vi "START ADD ITEM.vi"(10 "REFERENCES":T2, 11 "ITEM DATA IN":T1) -> (3 "ITEM DATA OUT":T1)   [LabVIEW 2019]
uses:
  Controls/References Cluster.ctl
  <vilib>/userDefined/High Color/IMAQdx.ctl
  Controls/Custom Calendar/Custom Calendar.xctl
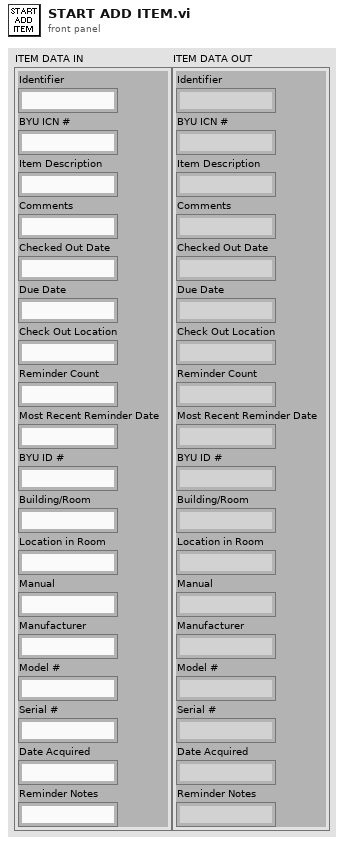
[diagram p1: front panel]
types:
  T1 = cluster{"Identifier":string, "BYU ICN #":string, "Item Description":string, "Comments":string, "Checked Out Date":string, "Due Date":string, "Check Out Location":string, "Reminder Count":string, "Most Recent Reminder Date":string, "BYU ID #":string, "Building/Room":string, "Location in Room":string, "Manual":string, "Manufacturer":string, "Model #":string, "Serial #":string, "Date Acquired":string, "Reminder Notes":string}
  T2 = typedef "References Cluster.ctl" = cluster{"MAIN PAGES":refnum<vi>, "ADD/EDIT ITEM REFERENCES":cluster{"Identifier":refnum<vi>, "BYU ICN #":refnum<vi>, "Item Description":refnum<vi>, "Comments":refnum<vi>, "Checked Out Date":refnum<vi>, "Due Date":refnum<vi>, "Check Out Location":refnum<vi>, "Reminder Count":refnum<vi>, "Most Recent Reminder Date":refnum<vi>, "BYU ID #":refnum<vi>, "Building/Room":refnum<vi>, "Location in Room":refnum<vi>, "Manual":refnum<vi>, "Manufacturer":refnum<vi>, "Model #":refnum<vi>, "Serial #":refnum<vi>, "Date Acquired":refnum<vi>, "ADD/EDIT ITEM LABEL":refnum<vi>, "ARCHIVE ITEM":refnum<vi>, "Archive Item Inputs":refnum<vi>, "Reminder Notes":refnum<vi>, "DUPLICATE ITEM":refnum<vi>}, "ADD/EDIT USER REFERENCES":cluster{"BYU ID # (##-###-####)":refnum<vi>, "First Name":refnum<vi>, "Last Name":refnum<vi>, "Phone Number (###-###-####)":refnum<vi>, "Email":refnum<vi>, "Department":refnum<vi>, "Graduation Status":refnum<vi>, "Anticipated Graduation Year":refnum<vi>, "Credit Score":refnum<vi>, "Date Added":refnum<vi>, "Graduation Clearance Date":refnum<vi>, "Picture File Name":refnum<vi>, "ADD/EDIT USER LABEL":refnum<vi>, "Department Map":refnum<vi>, "Status Map":refnum<vi>, "Anticipated Graduation Year Map":refnum<vi>, "User Agreement":refnum<vi>, "User Comments":refnum<vi>, "Camera":refnum<vi>}, "RETURN ITEM REFERENCES":cluster{"Item or Person:":refnum<vi>, "Search Return Results":refnum<vi>, "What are you searching for?":refnum<vi>}, "SEARCH DATABASE REFERENCES":cluster{"What to Search For:":refnum<vi>, "Where to Search":refnum<vi>, "Column to Search In":refnum<vi>, "Column to Sort By":refnum<vi>, "Search Database Results":refnum<vi>, "Inventory Column Selector":refnum<vi>, "User Column Selector":refnum<vi>, "Inventory Archive Column Selector":refnum<vi>, "User Archive Column Selector":refnum<vi>, "Sales Tracking Column Selector":refnum<vi>, "Checked In Archive Column Selector":refnum<vi>, "Restore User":refnum<vi>, "Date Range":refnum<vi>, "Dates Less Than":refnum<vi>, "Dates Greater Than":refnum<vi>, "Search Print Receipt":refnum<vi>, "Edit Sale Description":refnum<vi>}, "USER ITEMS REFERENCES":cluster{"USER'S INFORMATION":refnum<vi>, "User's Checked Out Items":refnum<vi>, "User Info Comments":refnum<vi>, "SEE USER INFO COMMENTS":refnum<vi>}, "EDIT ITEMS REFERENCES":cluster{"New Check Out Location":refnum<vi>, "Items to Edit":refnum<vi>, "Edit Items Due Date":refnum<vi>, "New Reminder Notes":refnum<vi>, "New Item Description":refnum<vi>}, "CHECK OUT ITEMS REFERENCES":cluster{"Enter Item:":refnum<vi>, "Check Out Items Due Date":refnum<vi>, "Check Out Location":refnum<vi>, "Items to be Checked Out":refnum<vi>, "Possible Items":refnum<vi>, "Altered Item Description":refnum<vi>}, "TRANSFER ITEMS REFERENCES":cluster{"Search Parameter":refnum<vi>, "What to Match":refnum<vi>, "Matching Individuals":refnum<vi>, "Items to be Transferred":refnum<vi>}, "SETTINGS REFERENCES":cluster{"PSC Database Settings":refnum<vi>, "PSC Sales Item Spreadsheet":refnum<vi>}, "PSC SALES REFERENCES":cluster{"BYU ID CARD #":refnum<vi>, "Sale Description":refnum<vi>, "Scan or Enter Item Name":refnum<vi>, "Items to be Sold":refnum<vi>, "Grand Total":refnum<vi>, "Item List":refnum<vi>}}
  T3 = enum32{"IDLE", "ADD/EDIT USER", "ADD/EDIT ITEM", "RETURN ITEMS", "SEARCH DATABASE", "USER ITEMS", "CHECK OUT ITEMS", "EDIT ITEMS", "TRANSFER ITEMS", "PSC SALES", "ATRIUM", "INVENTORY TRACKING", "SETTINGS"}
  T4 = cluster{"Identifier":refnum<vi>, "BYU ICN #":refnum<vi>, "Item Description":refnum<vi>, "Comments":refnum<vi>, "Checked Out Date":refnum<vi>, "Due Date":refnum<vi>, "Check Out Location":refnum<vi>, "Reminder Count":refnum<vi>, "Most Recent Reminder Date":refnum<vi>, "BYU ID #":refnum<vi>, "Building/Room":refnum<vi>, "Location in Room":refnum<vi>, "Manual":refnum<vi>, "Manufacturer":refnum<vi>, "Model #":refnum<vi>, "Serial #":refnum<vi>, "Date Acquired":refnum<vi>, "ADD/EDIT ITEM LABEL":refnum<vi>, "ARCHIVE ITEM":refnum<vi>, "Archive Item Inputs":refnum<vi>, "Reminder Notes":refnum<vi>, "DUPLICATE ITEM":refnum<vi>}
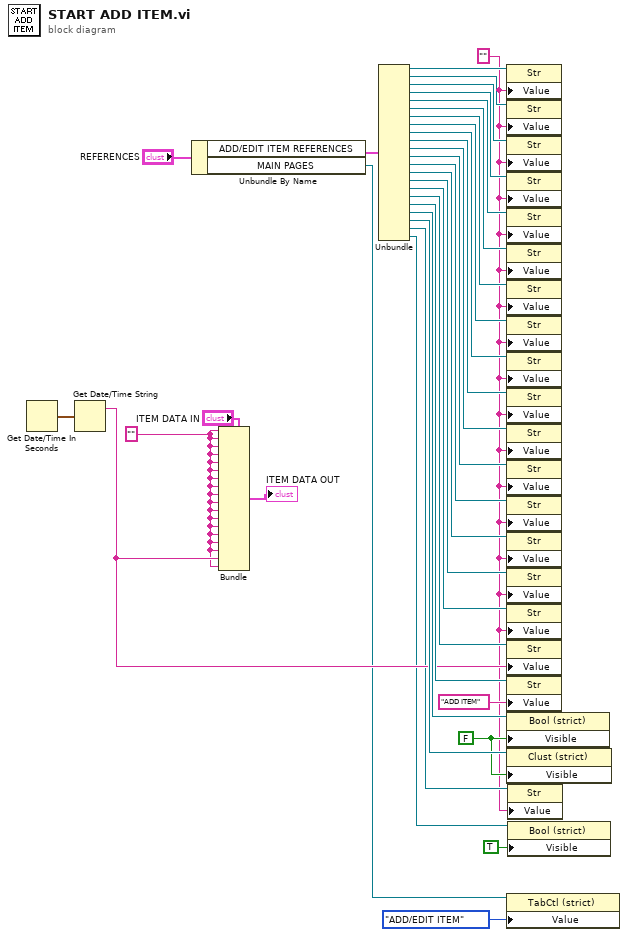
[diagram p0: block diagram]
diagram:
  w13 = FALSE ("Visible")
  w5 = "" ("BYU ID (##-###-####)")
  w3 = "" ("BYU ID (##-###-####)")
  n1 = Get Date/Time In Seconds() -> (seconds since 1Jan1904=w35:timestamp)
  n2 = Get Date/Time String(seconds (now)=w35) -> (date string=w8:string)  [unwired: 2 in, 1 out]
  n3 = Unbundle By Name("REFERENCES") -> ("ADD/EDIT ITEM REFERENCES"=w11:T4, "MAIN PAGES"=w7:refnum<vi>)
  n4 = Bundle(cluster="ITEM DATA IN", "Identifier"=w5, "BYU ICN #"=w5, "Item Description"=w5, "Comments"=w5, "Checked Out Date"=w5, "Due Date"=w5, "Check Out Location"=w5, "Reminder Count"=w5, "Most Recent Reminder Date"=w5, "BYU ID #"=w5, "Building/Room"=w5, "Location in Room"=w5, "Manual"=w5, "Manufacturer"=w5, "Model #"=w5, "Serial #"=w5, "Date Acquired"=w8, "Reminder Notes"=w5) -> (→"ITEM DATA OUT":T1)
  n5 = Unbundle(w11) -> ("Identifier"=w34:refnum<vi>, "BYU ICN #"=w33:refnum<vi>, "Item Description"=w32:refnum<vi>, "Comments"=w31:refnum<vi>, "Checked Out Date"=w30:refnum<vi>, "Due Date"=w29:refnum<vi>, "Check Out Location"=w28:refnum<vi>, "Reminder Count"=w27:refnum<vi>, "Most Recent Reminder Date"=w26:refnum<vi>, "BYU ID #"=w25:refnum<vi>, "Building/Room"=w24:refnum<vi>, "Location in Room"=w23:refnum<vi>, "Manual"=w22:refnum<vi>, "Manufacturer"=w21:refnum<vi>, "Model #"=w20:refnum<vi>, "Serial #"=w19:refnum<vi>, "Date Acquired"=w18:refnum<vi>, "ADD/EDIT ITEM LABEL"=w17:refnum<vi>, "ARCHIVE ITEM"=w15:refnum<vi>, "Archive Item Inputs"=w14:refnum<vi>, "Reminder Notes"=w4:refnum<vi>, "DUPLICATE ITEM"=w2:refnum<vi>)
  n6 = property class="Str"(reference=w34, "Value"=w3) -> ()  [unwired: 1 in, 2 out]
  n7 = property class="Str"(reference=w33, "Value"=w3) -> ()  [unwired: 1 in, 2 out]
  n8 = property class="Str"(reference=w32, "Value"=w3) -> ()  [unwired: 1 in, 2 out]
  n9 = property class="Str"(reference=w31, "Value"=w3) -> ()  [unwired: 1 in, 2 out]
  n10 = property class="Str"(reference=w30, "Value"=w3) -> ()  [unwired: 1 in, 2 out]
  n11 = property class="Str"(reference=w29, "Value"=w3) -> ()  [unwired: 1 in, 2 out]
  n12 = property class="Str"(reference=w28, "Value"=w3) -> ()  [unwired: 1 in, 2 out]
  n13 = property class="Str"(reference=w27, "Value"=w3) -> ()  [unwired: 1 in, 2 out]
  n14 = property class="Str"(reference=w26, "Value"=w3) -> ()  [unwired: 1 in, 2 out]
  n15 = property class="Str"(reference=w25, "Value"=w3) -> ()  [unwired: 1 in, 2 out]
  n16 = property class="Str"(reference=w24, "Value"=w3) -> ()  [unwired: 1 in, 2 out]
  n17 = property class="Str"(reference=w23, "Value"=w3) -> ()  [unwired: 1 in, 2 out]
  n18 = property class="Str"(reference=w22, "Value"=w3) -> ()  [unwired: 1 in, 2 out]
  n19 = property class="Str"(reference=w21, "Value"=w3) -> ()  [unwired: 1 in, 2 out]
  n20 = property class="Str"(reference=w20, "Value"=w3) -> ()  [unwired: 1 in, 2 out]
  n21 = property class="Str"(reference=w19, "Value"=w3) -> ()  [unwired: 1 in, 2 out]
  n22 = property class="Str"(reference=w18, "Value"=w8) -> ()  [unwired: 1 in, 2 out]
  n23 = property class="Str"(reference=w17, "Value"="ADD ITEM" ("ADD/EDIT ITEM LABEL")) -> ()  [unwired: 1 in, 2 out]
  n24 = property class="Bool (strict)"(reference=w15, "Visible"=w13) -> ()  [unwired: 1 in, 2 out]
  n25 = property class="Clust (strict)"(reference=w14, "Visible"=w13) -> ()  [unwired: 1 in, 2 out]
  n26 = property class="TabCtl (strict)"(reference=w7, "Value"=T3."ADD/EDIT ITEM") -> ()  [unwired: 1 in, 2 out]
  n27 = property class="Str"(reference=w4, "Value"=w3) -> ()  [unwired: 1 in, 2 out]
  n28 = property class="Bool (strict)"(reference=w2, "Visible"=TRUE) -> ()  [unwired: 1 in, 2 out]
